vi "runController.vi"(8 "error in (no error)":errorcluster, 11 "Boot in":refnum<class "Boot.lvclass">) -> (0 "error out":errorcluster, 3 "Boot out":refnum<class "Boot.lvclass">)   [LabVIEW 2016, in "Boot.lvclass"]
uses:
  Boot.lvclass
  Controller/Controller.lvclass
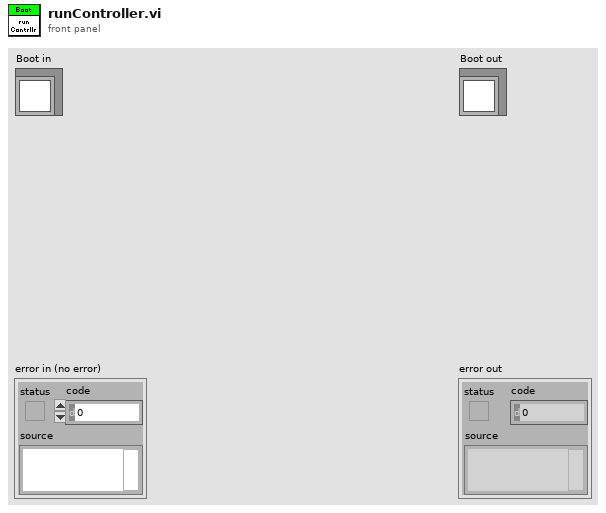
[diagram p1: front panel]
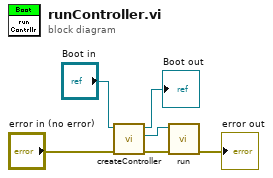
[diagram p0: block diagram]
diagram:
  n1 = call "createController.vi"("error in (no error)"="error in (no error)", "Boot in"="Boot in") -> ("error out"=w1:errorcluster, "Controller"=w4:refnum<class "Controller.lvclass">, "Boot out"=→"Boot out":refnum<class "Boot.lvclass">)  [unwired: 7 in]
  n2 = call "run.vi"("error in (no error)"=w1, "Controller in"=w4) -> ("error out"=→"error out":errorcluster)  [unwired: 8 in, 1 out]
